vi "get index definition.vi"(10 "channel classification":T1, 11 "GPIC Core configuration in":refnum<class "GPIC Core configuration.lvclass">) -> (1 "valid?":bool, 2 "index cluster":variant, 3 "GPIC Core configuration out":refnum<class "GPIC Core configuration.lvclass">)   [LabVIEW 2017, in "GPIC Core configuration.lvclass"]
uses:
  GPIC Core configuration.lvclass
  <vilib>/NI/Tag Bus Module Framework/channel/channel classification.ctl
  input data indices.ctl
  output data indices.ctl
  parameter data indices.ctl
  result data indices.ctl
  <vilib>/NI/Tag Bus Module Framework/channel/TBM channel.lvclass
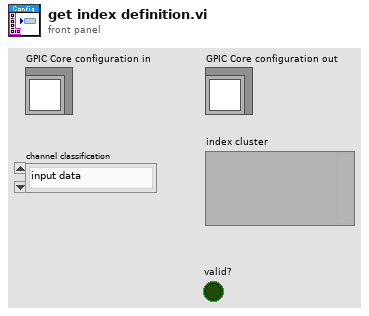
[diagram p1: front panel]
types:
  T1 = typedef "TBM channel.lvclass/channel classification.ctl" = enum16{"input data", "output data", "processing parameter", "processing result"}
  T2 = typedef "GPIC Core configuration.lvclass/input data indices.ctl" = cluster{"I16.AO_AO0":i32, "I16.AO_AO1":i32, "I16.AO_AO2":i32, "I16.AO_AO3":i32, "I16.AO_AO4":i32, "I16.AO_AO5":i32, "I16.AO_AO6":i32, "I16.AO_AO7":i32, "Boolean.HalfBridge_DO0":i32, "Boolean.HalfBridge_DO1":i32, "Boolean.HalfBridge_DO2":i32, "Boolean.HalfBridge_DO3":i32, "Boolean.HalfBridge_DO4":i32, "Boolean.HalfBridge_DO5":i32, "Boolean.HalfBridge_DO6":i32, "Boolean.HalfBridge_DO7":i32, "Boolean.HalfBridge_DO8":i32, "Boolean.HalfBridge_DO9":i32, "Boolean.HalfBridge_DO10":i32, "Boolean.HalfBridge_DO11":i32, "Boolean.HalfBridge_DO12":i32, "Boolean.HalfBridge_DO13":i32, "Boolean.LVTTL_DIO0":i32, "Boolean.LVTTL_DIO1":i32, "Boolean.LVTTL_DIO2":i32, "Boolean.LVTTL_DIO3":i32, "Boolean.LVTTL_DIO4":i32, "Boolean.LVTTL_DIO5":i32, "Boolean.LVTTL_DIO6":i32, "Boolean.LVTTL_DIO7":i32, "Boolean.LVTTL_DIO8":i32, "Boolean.LVTTL_DIO9":i32, "Boolean.LVTTL_DIO10":i32, "Boolean.LVTTL_DIO11":i32, "Boolean.LVTTL_DIO12":i32, "Boolean.LVTTL_DIO13":i32, "Boolean.LVTTL_DIO14":i32, "Boolean.LVTTL_DIO15":i32, "Boolean.LVTTL_DIO16":i32, "Boolean.LVTTL_DIO17":i32, "Boolean.LVTTL_DIO18":i32, "Boolean.LVTTL_DIO19":i32, "Boolean.LVTTL_DIO20":i32, "Boolean.LVTTL_DIO21":i32, "Boolean.LVTTL_DIO22":i32, "Boolean.LVTTL_DIO23":i32, "Boolean.LVTTL_DIO24":i32, "Boolean.LVTTL_DIO25":i32, "Boolean.LVTTL_DIO26":i32, "Boolean.LVTTL_DIO27":i32, "Boolean.LVTTL_DIO28":i32, "Boolean.LVTTL_DIO29":i32, "Boolean.LVTTL_DIO30":i32, "Boolean.LVTTL_DIO31":i32, "Boolean.RelayControl_DO0":i32, "Boolean.RelayControl_DO1":i32, "Boolean.RelayContro_DOl2":i32, "Boolean.RelayControl_DO3":i32, "Single.Scanned_AI0":i32, "Single.Scanned_AI1":i32, "Single.Scanned_AI2":i32, "Single.Scanned_AI3":i32, "Single.Scanned_AI4":i32, "Single.Scanned_AI5":i32, "Single.Scanned_AI6":i32, "Single.Scanned_AI7":i32, "Single.Simultaneous_AI0":i32, "Single.Simultaneous_AI1":i32, "Single.Simultaneous_AI2":i32, "Single.Simultaneous_AI3":i32, "Single.Simultaneous_AI4":i32, "Single.Simultaneous_AI5":i32, "Single.Simultaneous_AI6":i32, "Single.Simultaneous_AI7":i32, "Single.Simultaneous_AI8":i32, "Single.Simultaneous_AI9":i32, "Single.Simultaneous_AI10":i32, "Single.Simultaneous_AI11":i32, "Single.Simultaneous_AI12":i32, "Single.Simultaneous_AI13":i32, "Single.Simultaneous_AI14":i32, "Single.Simultaneous_AI15":i32, "Boolean.Sinking_DO0":i32, "Boolean.Sinking_DO1":i32, "Boolean.Sinking_DO2":i32, "Boolean.Sinking_DO3":i32, "Boolean.Sinking_DO4":i32, "Boolean.Sinking_DO5":i32, "Boolean.Sinking_DO6":i32, "Boolean.Sinking_DO7":i32, "Boolean.Sinking_DO8":i32, "Boolean.Sinking_DO9":i32, "Boolean.Sinking_DO10":i32, "Boolean.Sinking_DO11":i32, "Boolean.Sinking_DO12":i32, "Boolean.Sinking_DO13":i32, "Boolean.Sinking_DO14":i32, "Boolean.Sinking_DO15":i32, "Boolean.Sinking_DO16":i32, "Boolean.Sinking_DO17":i32, "Boolean.Sinking_DO18":i32, "Boolean.Sinking_DO19":i32, "Boolean.Sinking_DO20":i32, "Boolean.Sinking_DO21":i32, "Boolean.Sinking_DO22":i32, "Boolean.Sinking_DO23":i32, "Boolean.Sourcing_P0_DI0":i32, "Boolean.Sourcing_P0_DI1":i32, "Boolean.Sourcing_P0_DI2":i32, "Boolean.Sourcing_P0_DI3":i32, "Boolean.Sourcing_P0_DI4":i32, "Boolean.Sourcing_P0_DI5":i32, "Boolean.Sourcing_P0_DI6":i32, "Boolean.Sourcing_P0_DI7":i32, "Boolean.Sourcing_P0_DI8":i32, "Boolean.Sourcing_P0_DI9":i32, "Boolean.Sourcing_P0_DI10":i32, "Boolean.Sourcing_P0_DI11":i32, "Boolean.Sourcing_P0_DI12":i32, "Boolean.Sourcing_P0_DI13":i32, "Boolean.Sourcing_P1_DI0":i32, "Boolean.Sourcing_P1_DI1":i32, "Boolean.Sourcing_P1_DI2":i32, "Boolean.Sourcing_P1_DI3":i32, "Boolean.Sourcing_P1_DI4":i32, "Boolean.Sourcing_P1_DI5":i32, "Boolean.Sourcing_P1_DI6":i32, "Boolean.Sourcing_P1_DI7":i32, "Boolean.Sourcing_P1_DI8":i32, "Boolean.Sourcing_P1_DI9":i32, "Boolean.Sourcing_P1_DI10":i32, "Boolean.Sourcing_P1_DI11":i32, "Boolean.Sourcing_P1_DI12":i32, "Boolean.Sourcing_P1_DI13":i32}
  T3 = typedef "GPIC Core configuration.lvclass/output data indices.ctl" = cluster{"fmwk_placeholder":i32}
  T4 = typedef "GPIC Core configuration.lvclass/parameter data indices.ctl" = cluster{"fmwk_placeholder":i32}
  T5 = typedef "GPIC Core configuration.lvclass/result data indices.ctl" = cluster{"fmwk_placeholder":i32}
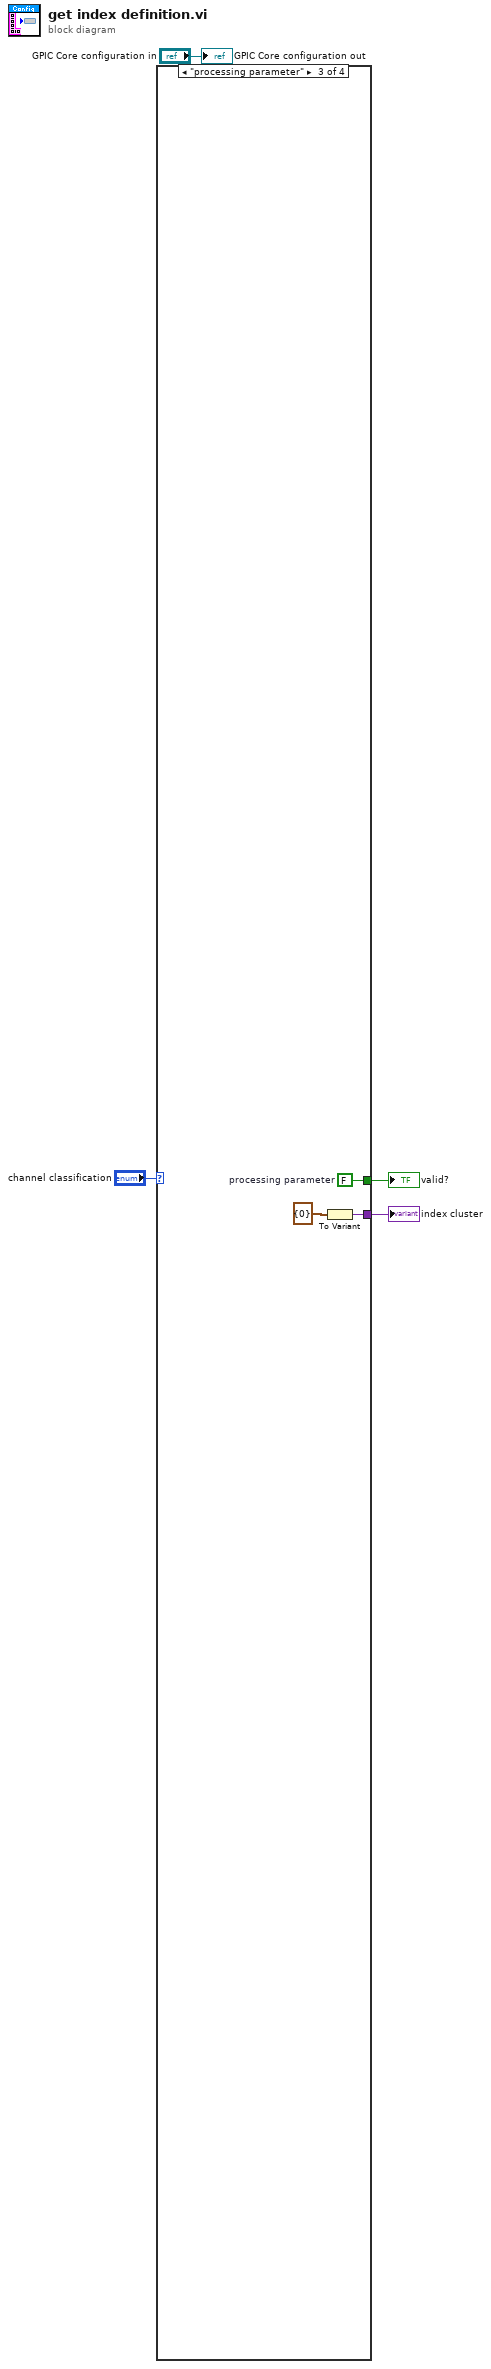
[diagram p0: block diagram]
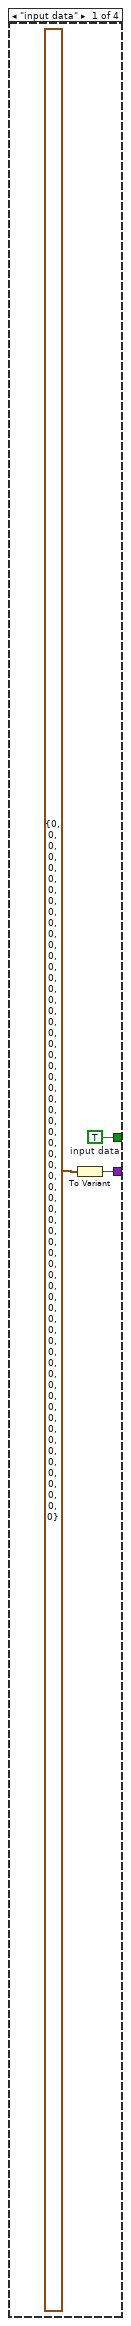
[diagram p2: hidden frame]
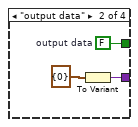
[diagram p3: hidden frame]
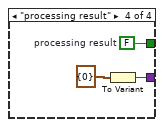
[diagram p4: hidden frame]
diagram:
  n1 = case shown="\"processing parameter\"" "channel classification" {
    tunnel: [w6 w10 w13 w16] -> w2
    tunnel: [w5 w9 w12 w15] -> w1
    frame "input data" {
      w5 = TRUE  # input data
      n2 = To Variant(anything=T2 {"I16.AO_AO0"=0, "I16.AO_AO1"=0, "I16.AO_AO2"=0, "I16.AO_AO3"=0, "I16.AO_AO4"=0, "I16.AO_AO5"=0, "I16.AO_AO6"=0, "I16.AO_AO7"=0, "Boolean.HalfBridge_DO0"=0, "Boolean.HalfBridge_DO1"=0, "Boolean.HalfBridge_DO2"=0, "Boolean.HalfBridge_DO3"=0, "Boolean.HalfBridge_DO4"=0, "Boolean.HalfBridge_DO5"=0, "Boolean.HalfBridge_DO6"=0, "Boolean.HalfBridge_DO7"=0, "Boolean.HalfBridge_DO8"=0, "Boolean.HalfBridge_DO9"=0, "Boolean.HalfBridge_DO10"=0, "Boolean.HalfBridge_DO11"=0, "Boolean.HalfBridge_DO12"=0, "Boolean.HalfBridge_DO13"=0, "Boolean.LVTTL_DIO0"=0, "Boolean.LVTTL_DIO1"=0, "Boolean.LVTTL_DIO2"=0, "Boolean.LVTTL_DIO3"=0, "Boolean.LVTTL_DIO4"=0, "Boolean.LVTTL_DIO5"=0, "Boolean.LVTTL_DIO6"=0, "Boolean.LVTTL_DIO7"=0, "Boolean.LVTTL_DIO8"=0, "Boolean.LVTTL_DIO9"=0, "Boolean.LVTTL_DIO10"=0, "Boolean.LVTTL_DIO11"=0, "Boolean.LVTTL_DIO12"=0, "Boolean.LVTTL_DIO13"=0, "Boolean.LVTTL_DIO14"=0, "Boolean.LVTTL_DIO15"=0, "Boolean.LVTTL_DIO16"=0, "Boolean.LVTTL_DIO17"=0, "Boolean.LVTTL_DIO18"=0, "Boolean.LVTTL_DIO19"=0, "Boolean.LVTTL_DIO20"=0, "Boolean.LVTTL_DIO21"=0, "Boolean.LVTTL_DIO22"=0, "Boolean.LVTTL_DIO23"=0, "Boolean.LVTTL_DIO24"=0, "Boolean.LVTTL_DIO25"=0, "Boolean.LVTTL_DIO26"=0, "Boolean.LVTTL_DIO27"=0, "Boolean.LVTTL_DIO28"=0, "Boolean.LVTTL_DIO29"=0, "Boolean.LVTTL_DIO30"=0, "Boolean.LVTTL_DIO31"=0, "Boolean.RelayControl_DO0"=0, "Boolean.RelayControl_DO1"=0, "Boolean.RelayContro_DOl2"=0, "Boolean.RelayControl_DO3"=0, "Single.Scanned_AI0"=0, "Single.Scanned_AI1"=0, "Single.Scanned_AI2"=0, "Single.Scanned_AI3"=0, "Single.Scanned_AI4"=0, "Single.Scanned_AI5"=0, "Single.Scanned_AI6"=0, "Single.Scanned_AI7"=0, "Single.Simultaneous_AI0"=0, "Single.Simultaneous_AI1"=0, "Single.Simultaneous_AI2"=0, "Single.Simultaneous_AI3"=0, "Single.Simultaneous_AI4"=0, "Single.Simultaneous_AI5"=0, "Single.Simultaneous_AI6"=0, "Single.Simultaneous_AI7"=0, "Single.Simultaneous_AI8"=0, "Single.Simultaneous_AI9"=0, "Single.Simultaneous_AI10"=0, "Single.Simultaneous_AI11"=0, "Single.Simultaneous_AI12"=0, "Single.Simultaneous_AI13"=0, "Single.Simultaneous_AI14"=0, "Single.Simultaneous_AI15"=0, "Boolean.Sinking_DO0"=0, "Boolean.Sinking_DO1"=0, "Boolean.Sinking_DO2"=0, "Boolean.Sinking_DO3"=0, "Boolean.Sinking_DO4"=0, "Boolean.Sinking_DO5"=0, "Boolean.Sinking_DO6"=0, "Boolean.Sinking_DO7"=0, "Boolean.Sinking_DO8"=0, "Boolean.Sinking_DO9"=0, "Boolean.Sinking_DO10"=0, "Boolean.Sinking_DO11"=0, "Boolean.Sinking_DO12"=0, "Boolean.Sinking_DO13"=0, "Boolean.Sinking_DO14"=0, "Boolean.Sinking_DO15"=0, "Boolean.Sinking_DO16"=0, "Boolean.Sinking_DO17"=0, "Boolean.Sinking_DO18"=0, "Boolean.Sinking_DO19"=0, "Boolean.Sinking_DO20"=0, "Boolean.Sinking_DO21"=0, "Boolean.Sinking_DO22"=0, "Boolean.Sinking_DO23"=0, "Boolean.Sourcing_P0_DI0"=0, "Boolean.Sourcing_P0_DI1"=0, "Boolean.Sourcing_P0_DI2"=0, "Boolean.Sourcing_P0_DI3"=0, "Boolean.Sourcing_P0_DI4"=0, "Boolean.Sourcing_P0_DI5"=0, "Boolean.Sourcing_P0_DI6"=0, "Boolean.Sourcing_P0_DI7"=0, "Boolean.Sourcing_P0_DI8"=0, "Boolean.Sourcing_P0_DI9"=0, "Boolean.Sourcing_P0_DI10"=0, "Boolean.Sourcing_P0_DI11"=0, "Boolean.Sourcing_P0_DI12"=0, "Boolean.Sourcing_P0_DI13"=0, "Boolean.Sourcing_P1_DI0"=0, "Boolean.Sourcing_P1_DI1"=0, "Boolean.Sourcing_P1_DI2"=0, "Boolean.Sourcing_P1_DI3"=0, "Boolean.Sourcing_P1_DI4"=0, "Boolean.Sourcing_P1_DI5"=0, "Boolean.Sourcing_P1_DI6"=0, "Boolean.Sourcing_P1_DI7"=0, "Boolean.Sourcing_P1_DI8"=0, "Boolean.Sourcing_P1_DI9"=0, "Boolean.Sourcing_P1_DI10"=0, "Boolean.Sourcing_P1_DI11"=0, "Boolean.Sourcing_P1_DI12"=0, "Boolean.Sourcing_P1_DI13"=0} ("Cluster")) -> (Variant=w6:variant)
    }
    frame "output data" {
      w9 = FALSE  # output data
      n3 = To Variant(anything=T3 {"fmwk_placeholder"=0} ("Cluster")) -> (Variant=w10:variant)
    }
    frame "processing parameter" {
      w12 = FALSE  # processing parameter
      n4 = To Variant(anything=T4 {"fmwk_placeholder"=0} ("Cluster")) -> (Variant=w13:variant)
    }
    frame "processing result" {
      w15 = FALSE  # processing result
      n5 = To Variant(anything=T5 {"fmwk_placeholder"=0} ("Cluster")) -> (Variant=w16:variant)
    }
  }
  "index cluster" <- w2
  "valid?" <- w1
  "GPIC Core configuration out" <- "GPIC Core configuration in"
